vi "Lockout state.vi"(8 "error in (no error)":errorcluster, 10 "Initial indicator states in":T2 {"Time Count" format="%.2g"}, 11 "Runtime statuses in":T1) -> (0 "error out":errorcluster, 2 "Initial indicator states out":T2 {"Time Count" format="%.2g"}, 3 "Runtime statuses out":T1)   [LabVIEW 2014]
doc: "Sets Boiler Status values and Runtime status values to values for \"Lockout\" state"
uses:
  Controls/Boiler Status Indicators.ctl
  Controls/Boiler runtime status indicators.ctl
  Controls/Log file FGV action enum.ctl
  Controls/Log event enum.ctl
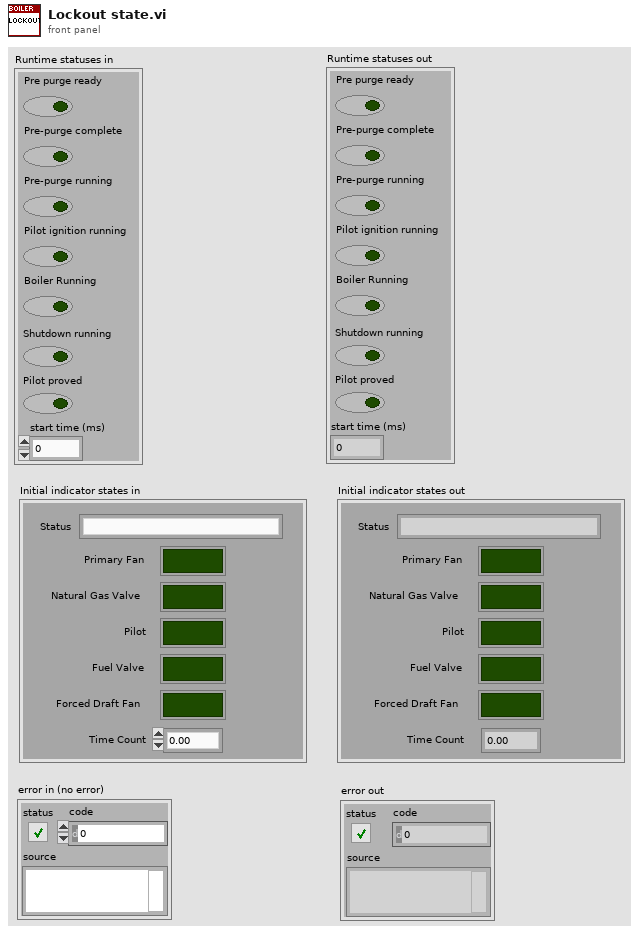
[diagram p1: front panel]
types:
  T1 = typedef "Boiler runtime status indicators.ctl" = cluster{"Pre purge ready":bool, "Pre-purge complete":bool, "Pre-purge running":bool, "Pilot ignition running":bool, "Boiler Running":bool, "Shutdown running":bool, "Pilot proved":bool, "start time (ms)":u32}
  T2 = typedef "Boiler Status Indicators.ctl" = cluster{"Status":string, "Primary Fan":bool, "Natural Gas Valve":bool, "Pilot":bool, "Fuel Valve":bool, "Forced Draft Fan":bool, "Time Count":dbl}
  T3 = typedef "Log event enum.ctl" = enum16{"Boiler Initialized", "Boiler Ready", "Start Pre-Purge", "Pre-Purge Complete", "Pilot ON", "Pilot proved", "Forced Draft Fan ON", "Boiler Running", "Start Shutdown Purge", "Shutdown Purge Complete"}
  T4 = typedef "Log file FGV action enum.ctl" = enum16{"open log file", "log event", "close log file"}
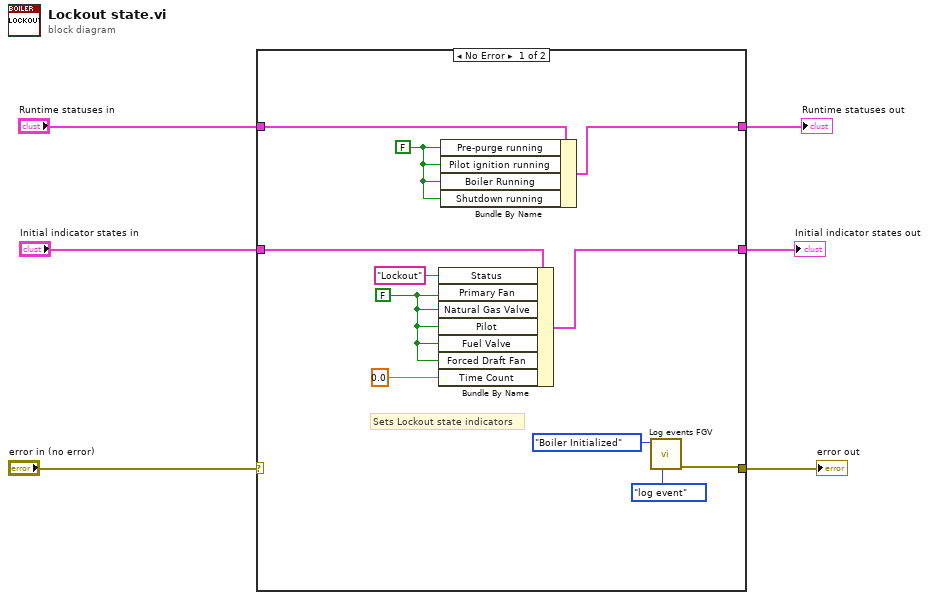
[diagram p0: block diagram]
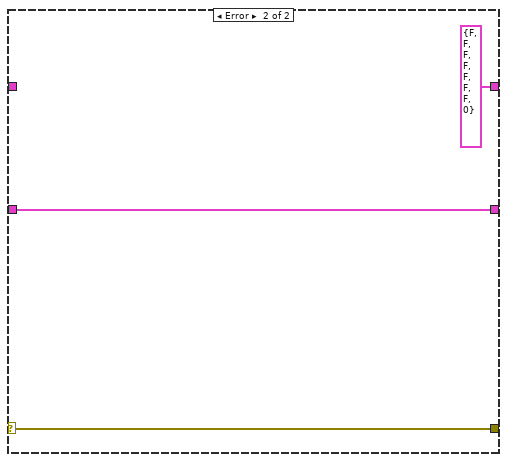
[diagram p2: hidden frame]
diagram:
  n1 = case shown="No Error" "error in (no error)" {
    selector: "error in (no error)" -> [_ w20]
    tunnel: [w17 w19] -> w6
    tunnel: "Initial indicator states in" -> [w16 w19]
    tunnel: [w8 w20] -> w3
    tunnel: "Runtime statuses in" -> [w12 _]
    tunnel: [w11 T1 {"Pre purge ready"=FALSE, "Pre-purge complete"=FALSE, "Pre-purge running"=FALSE, "Pilot ignition running"=FALSE, "Boiler Running"=FALSE, "Shutdown running"=FALSE, "Pilot proved"=FALSE, "start time (ms)"=0} ("Runtime statuses in")] -> w1
    frame No Error {
      w10 = FALSE ("Pre-purge running")
      w13 = FALSE ("Primary Fan")
      # "Sets Lockout state indicators"
      n2 = Bundle By Name(cluster=w16, "Status"="Lockout", "Primary Fan"=w13, "Natural Gas Valve"=w13, "Pilot"=w13, "Fuel Valve"=w13, "Forced Draft Fan"=w13, "Time Count"=0.0) -> (w17:T2)
      n3 = Bundle By Name(cluster=w12, "Pre-purge running"=w10, "Pilot ignition running"=w10, "Boiler Running"=w10, "Shutdown running"=w10) -> (w11:T1)
      n4 = call "Log events FGV.vi"("action"=Log_file_FGV_action_enum."log event", "Log event"=Log_event_enum."Boiler Initialized") -> ("error out"=w8:errorcluster)  [unwired: 9 in]
    }
    frame Error {
    }
  }
  "Initial indicator states out" <- w6
  "error out" <- w3
  "Runtime statuses out" <- w1
